vi "Asylum_Interpolation.vi"(0 "X":dbl[](array[numeric]), 1 "Y":dbl[](array[numeric]), 2 "V":dbl[](array[numeric]), 3 "Interpolation":dbl format="%#_13g") -> (7 "X":dbl[](array[numeric]), 8 "Y":dbl[](array[numeric]), 9 "V":dbl[](array[numeric]))   [LabVIEW 2019]
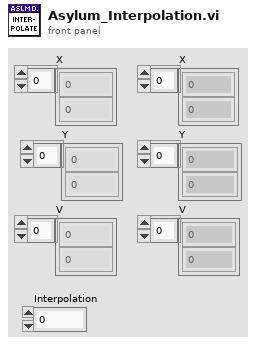
[diagram p1: front panel]
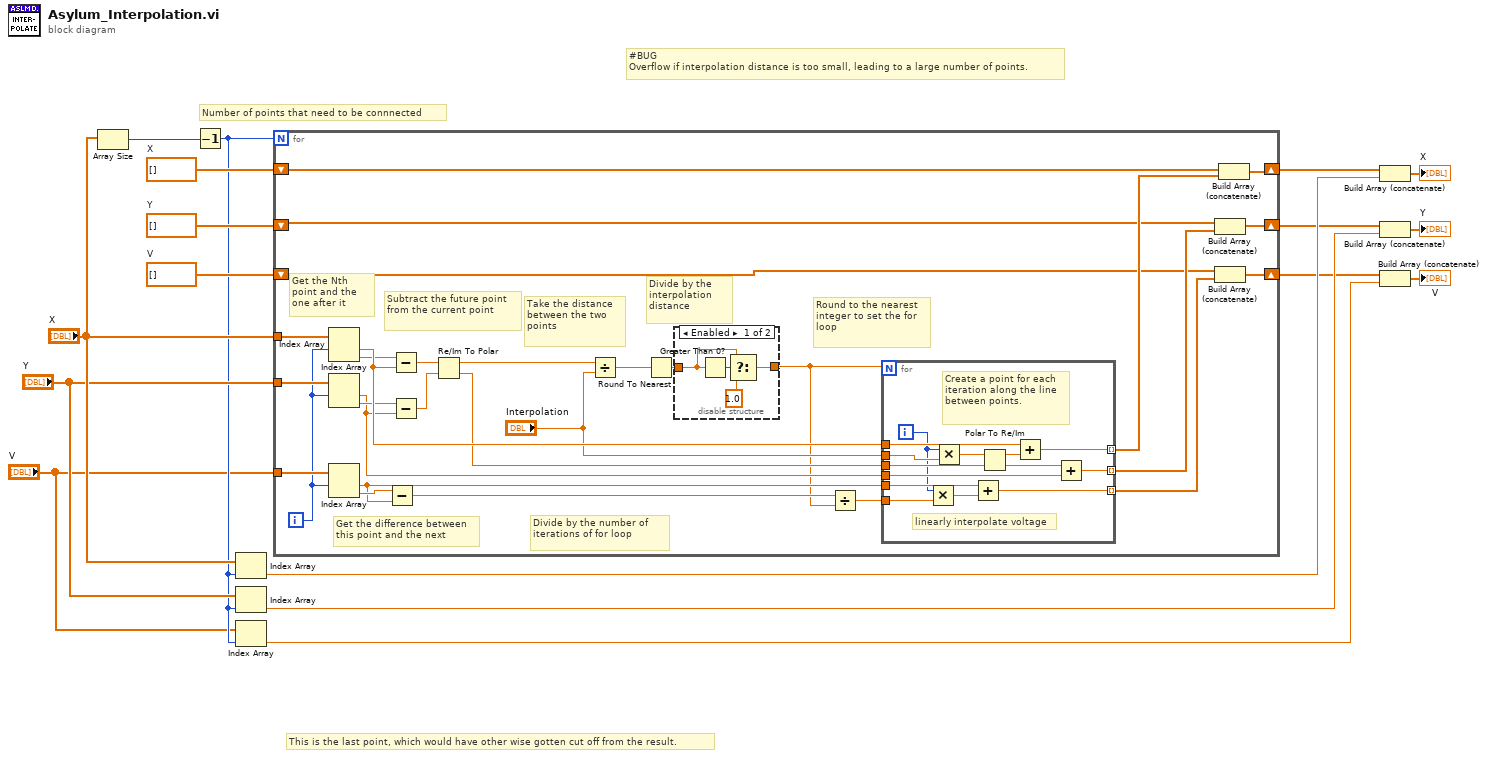
[diagram p0: block diagram]
diagram:
  w6 = dbl[] []  # V
  w12 = dbl[] []  # Y
  w13 = dbl[] []  # X
  # "#BUG\nOverflow if interpolation distance is too small, leading to a large number of points."
  # "This is the last point, which would have other wise gotten cut off from the result."
  # "Number of points that need to be connnected"
  n1 = Array Size(array="X") -> (size(s)=w14:i32)
  n2 = Decrement(x=w14) -> (x-1=w4:i32)
  n3 = Index Array(array="X", index=w4) -> (element=w16:dbl)
  n4 = Index Array(array="Y", index=w4) -> (element=w9:dbl)
  n5 = Index Array(array="V", index=w4) -> (element=w2:dbl)
  n6 = for {
    N: w4 -> [_]
    tunnel: "X" -> [w46]
    shift-right: [w41] -> w17
    shift-left: w13 -> [w40]
    tunnel: "Y" -> [w39]
    shift-right: [w33] -> w10
    shift-left: w12 -> [w32]
    tunnel: "V" -> [w30]
    shift-right: [w22] -> w5
    shift-left: w6 -> [w23]
    i -> [w29]
    # "Divide by the number of iterations of for loop"
    # "Get the difference between this point and the next"
    # "Subtract the future point from the current point"
    # "Get the Nth point and the one after it"
    # "Round to the nearest integer to set the for loop"
    # "Divide by the interpolation distance"
    # "Take the distance between the two points"
    n7 = Index Array(array=w46, index #1=w29) -> (element #1=w43:dbl, element #2=w42:dbl)  [unwired: 1 in]
    n8 = Index Array(array=w39, index #1=w29) -> (element #1=w35:dbl, element #2=w37:dbl)  [unwired: 1 in]
    n9 = Index Array(array=w30, index #1=w29) -> (element #1=w25:dbl, element #2=w28:dbl)  [unwired: 1 in]
    n10 = Subtract(x=w28, y=w25) -> (x-y=w27:dbl)
    n11 = Subtract(x=w42, y=w43) -> (x-y=w38:dbl)
    n12 = Subtract(x=w37, y=w35) -> (x-y=w36:dbl)
    n13 = Re/Im To Polar(2:w36, 3:w38) -> (0:w31:dbl, 1:w45:dbl)
    n14 = Divide(x=w45, y="Interpolation") -> (x/y=w44:dbl)
    n15 = Round To Nearest(number=w44) -> (nearest integer value=w20:dbl)
    n16 = disable-structure shown="Enabled" {
      disable-tunnel: w20 -> [w48 w51]
      disable-tunnel: [w47 w51] -> w18
      frame Enabled {
        n17 = Greater Than 0?(x=w48) -> (x > 0?=w50:bool)
        n18 = Select(t=w48, s=w50, f=1.0) -> (s? t:f=w47:dbl)
      }
      frame Disabled {
      }
    }
    n19 = Divide(x=w27, y=w18) -> (x/y=w26:dbl)
    n20 = for {
      N: w18 -> [_]
      tunnel: w43 -> [w57]
      tunnel: "Interpolation" -> [w58]
      tunnel: w31 -> [w64]
      tunnel: w35 -> [w60]
      tunnel: [w62] -> w24 mode=indexing
      tunnel: [w61] -> w34 mode=indexing
      tunnel: w26 -> [w52]
      tunnel: w25 -> [w55]
      tunnel: [w54] -> w21 mode=indexing
      i -> [w53]
      # "linearly interpolate voltage"
      # "Create a point for each iteration along the line between points."
      n21 = Multiply(x=w53, y=w52) -> (x*y=w56:dbl)
      n22 = Multiply(x=w53, y=w58) -> (x*y=w65:dbl)
      n23 = Add(x=w55, y=w56) -> (x+y=w54:dbl)
      n24 = Polar To Re/Im(2:w64, 3:w65) -> (0:w59:dbl, 1:w63:dbl)
      n25 = Add(x=w57, y=w63) -> (x+y=w61:dbl)
      n26 = Add(x=w59, y=w60) -> (x+y=w62:dbl)
    }
    n27 = Build Array (concatenate)(w32, w24) -> (w33:dbl[])
    n28 = Build Array (concatenate)(w23, w21) -> (w22:dbl[])
    n29 = Build Array (concatenate)(w40, w34) -> (w41:dbl[])
  }
  n30 = Build Array (concatenate)(w17, w16) -> (→"X":dbl[])
  n31 = Build Array (concatenate)(w10, w9) -> (→"Y":dbl[])
  n32 = Build Array (concatenate)(w5, w2) -> (→"V":dbl[])
